vi "Convert to Continuous.vi"(9 "Lower Limit Threshold":dbl=-180.0 format="%#_13g", 10 "Upper Limit Threshold":dbl=180.0 format="%#_13g", 11 "Input Value":dbl(knob) step=1.0 scale=-180.0..180.0) -> (2 "Continuous Value":dbl, 3 "Rollovers":dbl)   [LabVIEW 2018]
doc: "Converts a discontinous input value of a range into a continouous value. Must have discontinuity accross 0."
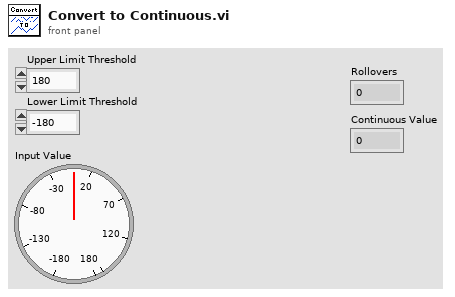
[diagram p1: front panel]
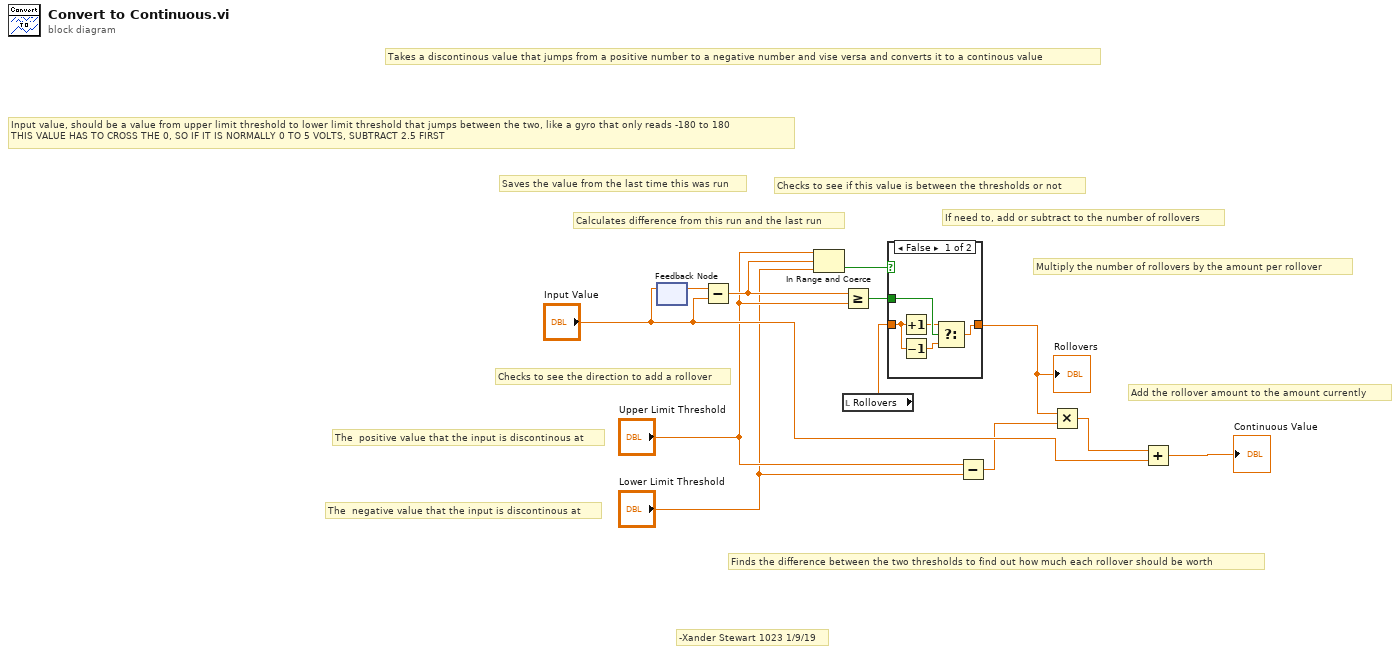
[diagram p0: block diagram]
diagram:
  # "-Xander Stewart 1023 1/9/19"
  # "Takes a discontinous value that jumps from a positive number to a negative number and vise versa and converts it to a continous value"
  # "If need to, add or subtract to the number of rollovers"
  # "Checks to see the direction to add a rollover"
  # "Add the rollover amount to the amount currently"
  # "Multiply the number of rollovers by the amount per rollover"
  # "Finds the difference between the two thresholds to find out how much each rollover should be worth"
  # "Checks to see if this value is between the thresholds or not"
  # "Calculates difference from this run and the last run"
  # "The  positive value that the input is discontinous at"
  # "The  negative value that the input is discontinous at"
  # "Saves the value from the last time this was run"
  # "Input value, should be a value from upper limit threshold to lower limit threshold that jumps between the two, like a gyro that only reads -180 to 180 \nTHIS VALUE HAS TO CROSS THE 0, SO IF IT IS NORMALLY 0 TO 5 VOLTS, SUBTRACT 2.5 FIRST"
  n1 = feedback-in #1("Input Value") -> ()
  n2 = feedback #1() -> (w12:dbl)  [unwired: 1 in]
  n3 = Subtract(x=w12, y="Input Value") -> (x-y=w11:dbl)
  n4 = In Range and Coerce(upper limit="Upper Limit Threshold", x=w11, lower limit="Lower Limit Threshold") -> (In Range?=w10:bool)  [unwired: 1 out]
  n5 = Greater Or Equal?(x=w11, y="Upper Limit Threshold") -> (x >= y?=w9:bool)
  n6 = local read "Rollovers"() -> (w4:dbl)
  n7 = case shown="False" w10 {
    tunnel: w4 -> [w17 w18]
    tunnel: [w16 w18] -> w5
    tunnel: w9 -> [w15 _]
    frame False {
      n8 = Increment(x=w17) -> (x+1=w14:dbl)
      n9 = Decrement(x=w17) -> (x-1=w13:dbl)
      n10 = Select(t=w14, s=w15, f=w13) -> (s? t:f=w16:dbl)
    }
    frame True {
    }
  }
  "Rollovers" <- w5
  n11 = Subtract(x="Upper Limit Threshold", y="Lower Limit Threshold") -> (x-y=w3:dbl)
  n12 = Multiply(x=w5, y=w3) -> (x*y=w8:dbl)
  n13 = Add(x=w8, y="Input Value") -> (x+y=→"Continuous Value":dbl)
